vi "Get Strings from Ref.vi"(8 "error in (no error)":errorcluster, 9 "Label Prefix":string, 10 "GObj Refnum in":refnum<vi>, 11 "DiagramText in":refnum<class "StringConstant.lvclass">) -> (0 "error out":errorcluster, 1 "Valid?":bool, 2 "GObj Refnum out":refnum<vi>, 3 "DiagramText out":refnum<class "StringConstant.lvclass">, 4 "GObj Name":string)   [LabVIEW 2013, in "SET Project Data.lvlib" / "StringConstant.lvclass"]
uses:
  StringConstant.lvclass
  GObject/GObject.lvclass/GObject.ctl
  GObject/Write Label.vi
  GObject/Write UID.vi
  GObject/Write ClassName.vi
  GObject/GObject.lvclass
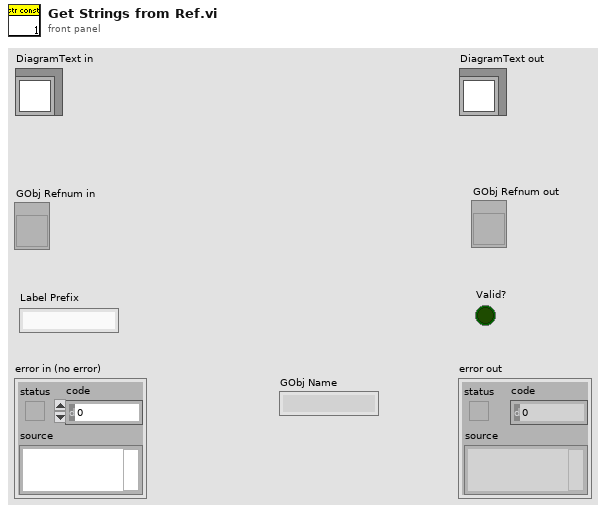
[diagram p1: front panel]
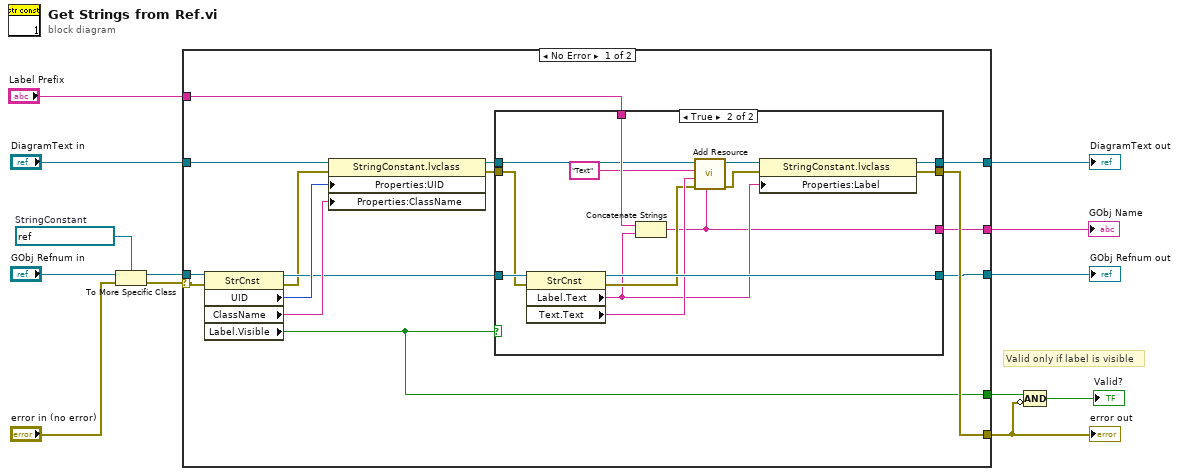
[diagram p0: block diagram]
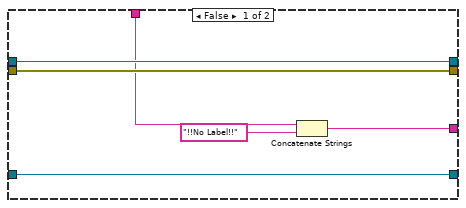
[diagram p2: hidden frame]
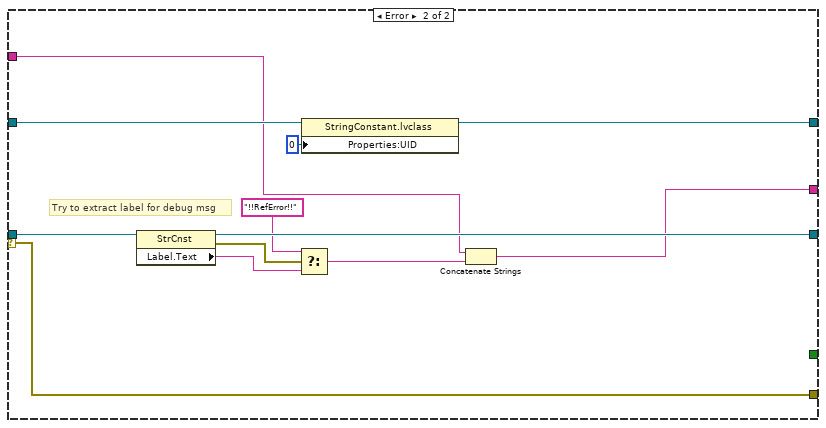
[diagram p3: hidden frame]
diagram:
  w11 = refnum<vi> refnum  # StringConstant
  # "Valid only if label is visible"
  n1 = To More Specific Class(target class=w11, reference="GObj Refnum in", error in="error in (no error)") -> (specific class reference=w9:refnum<vi>, error out=w10:errorcluster)
  n2 = case shown="No Error" w10 {
    selector: w10 -> [w21 w60]
    tunnel: w9 -> [w27 w56]
    tunnel: [w17 w55] -> w8
    tunnel: [w18 w60] -> w3
    tunnel: "DiagramText in" -> [w28 w59]
    tunnel: [w23 w57] -> w6
    tunnel: "Label Prefix" -> [w16 w50]
    tunnel: [w15 _] -> w4
    tunnel: [w14 w54] -> w1
    frame No Error {
      n3 = property class="StrCnst"(reference=w27, error in=w21) -> (reference out=w22:refnum<vi>, error out=w20:errorcluster, "UID"=w26:i32, "ClassName"=w25:string, "Label.Visible"=w15:bool)
      n4 = property class="StringConstant.lvclass"(reference=w28, error in=w20, "Properties:UID"=w26, "Properties:ClassName"=w25) -> (reference out=w24:refnum<class "StringConstant.lvclass">, error out=w19:errorcluster)
      n5 = case shown="True" w15 {
        tunnel: w24 -> [w34 w42]
        tunnel: [w34 w48] -> w23
        tunnel: w22 -> [w32 w47]
        tunnel: w19 -> [w33 w46]
        tunnel: [w33 w45] -> w18
        tunnel: [w32 w44] -> w17
        tunnel: w16 -> [w31 w43]
        tunnel: [w29 w35] -> w14
        frame False {
          n6 = Concatenate Strings(w31, "!!No Label!!") -> (w29:string)
        }
        frame True {
          n7 = property class="StrCnst"(reference=w47, error in=w46) -> (reference out=w44:refnum<vi>, error out=w38:errorcluster, "Label.Text"=w36:string, "Text.Text"=w39:string)
          n8 = Concatenate Strings(w43, w36) -> (w35:string)
          n9 = call "Add Resource.vi"("TagPrefix"=w35, "error in (no error)"=w38, "ItemText"=w39, "ItemName"="Text" ("name"), "GObject in"=w42) -> ("error out"=w37:errorcluster, "GObject out"=w41:refnum<class "StringConstant.lvclass">)  [unwired: 5 in]
          n10 = property class="StringConstant.lvclass"(reference=w41, error in=w37, "Properties:Label"=w36) -> (reference out=w48:refnum<class "StringConstant.lvclass">, error out=w45:errorcluster)
        }
      }
    }
    frame Error {
      # "Try to extract label for debug msg"
      n11 = property class="StrCnst"(reference=w56) -> (reference out=w55:refnum<vi>, error out=w53:errorcluster, "Label.Text"=w51:string)  [unwired: 1 in]
      n12 = Select(t="!!RefError!!" ("Label.Text"), s=w53, f=w51) -> (s? t:f=w49:string)
      n13 = property class="StringConstant.lvclass"(reference=w59, "Properties:UID"=0 ("UID")) -> (reference out=w57:refnum<class "StringConstant.lvclass">)  [unwired: 1 in, 1 out]
      n14 = Concatenate Strings(w50, w49) -> (w54:string)
    }
  }
  "error out" <- w3
  "DiagramText out" <- w6
  "GObj Refnum out" <- w8
  "GObj Name" <- w1
  n15 = Compound Arithmetic op=AND(w4, invert w3) -> (→"Valid?":bool)
